vi "ConveyorBelt_Create.vi"(0 "reference in":refnum<class "ConveyorBelt.lvclass">, 2 "ConveyorBeltRef":refnum<vi>, 5 "error in (no error)":errorcluster) -> (14 "reference out":refnum<class "ConveyorBelt.lvclass">, 19 "error out":errorcluster)   [LabVIEW 2014, in "ConveyorBelt.lvclass"]
uses:
  ConveyorBelt.lvclass
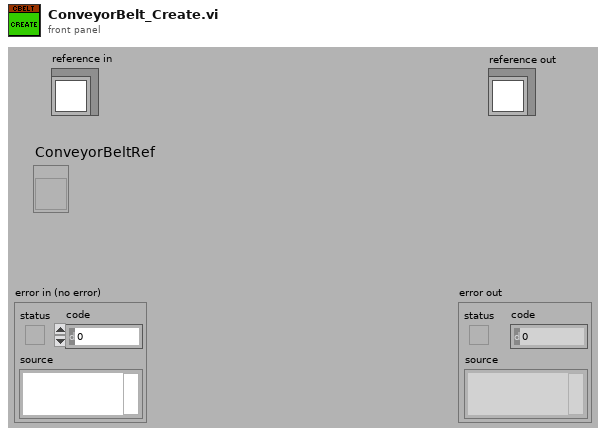
[diagram p1: front panel]
types:
  T1 = typedef "ConveyorBelt.lvclass/ObjectAttributes.ctl" = cluster{"Right":bool, "Running":bool, "ConveyorBeltRef":refnum<vi>}
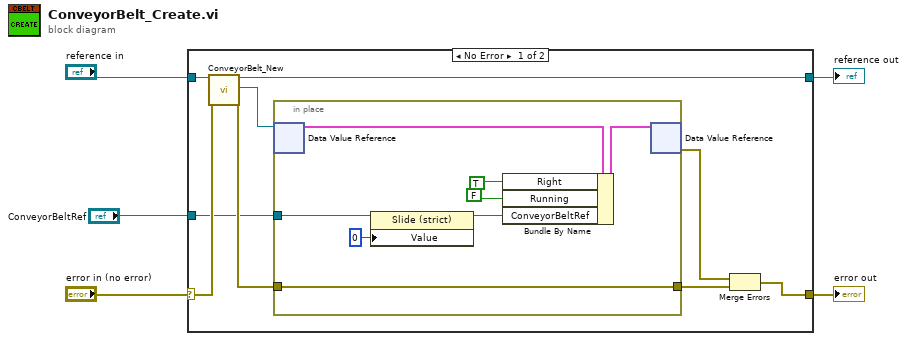
[diagram p0: block diagram]
diagram:
  n1 = case shown="No Error" "error in (no error)" {
    selector: "error in (no error)" -> [w13 w24]
    tunnel: [w10 w24] -> w4
    tunnel: "reference in" -> [w14 w23]
    tunnel: [w12 w23] -> w2
    tunnel: "ConveyorBeltRef" -> [w6 _]
    frame No Error {
      n2 = call "ConveyorBelt_New.vi"("reference in"=w14, "error in (no error)"=w13) -> ("reference out"=w12:refnum<class "ConveyorBelt.lvclass">, "DVRRefOut"=w9:refnum<data-value>, "error out"=w8:errorcluster)  [unwired: 14 in, 1 out]
      n3 = in-place {
        in-place-border: w8 -> [w20]
        in-place-border: [w20] -> w7
        in-place-border: w6 -> [w15]
        n4 = in-place-dvr #1(w9) -> (w21:T1)  [unwired: 1 out]
        n5 = property class="Slide (strict)"(reference=w15, "Value"=u8 0) -> (reference out=w16:refnum<vi>)  [unwired: 1 in, 1 out]
        n6 = Bundle By Name(cluster=w21, "Right"=TRUE ("None"), "Running"=FALSE, "ConveyorBeltRef"=w16) -> (w22:T1)
        n7 = in-place-dvr #1(w22) -> (w11:errorcluster)  [unwired: 1 out]
      }
      n8 = Merge Errors(w11, w7) -> (w10:errorcluster)
    }
    frame Error {
    }
  }
  "error out" <- w4
  "reference out" <- w2
